vi "国弘恢复出厂.vi"(7 "探头":u16(ring)=5 items=["NULL", "pH", "Cond", "DO", "Turb", "ORP", "6", "7", "8", "9", "氯化物"], 8 "error in (no error)":errorcluster caption="错误输入（无错误）") -> (0 "error out":errorcluster caption="错误输出", 3 "MB session out":refnum<class "MB_Master.lvclass">)   [LabVIEW 2022 SP3, in "斯坦道多参数.lvlib"]
uses:
  <vilib>/Plasmionique/MB Master/MB_Master/MB_Master.lvclass
  <vilib>/Plasmionique/MB Master/MB Master.lvlib
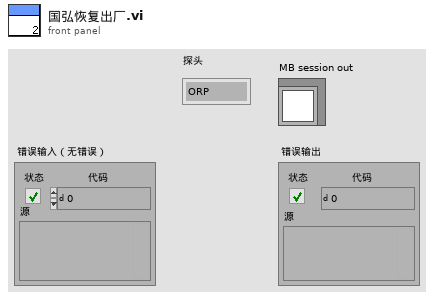
[diagram p1: front panel]
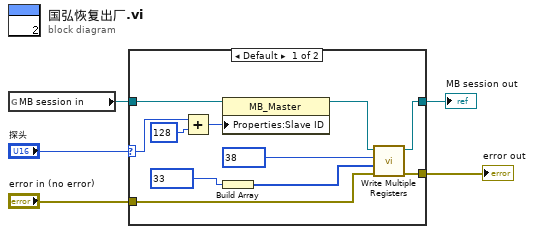
[diagram p0: block diagram]
diagram:
  n1 = global read "多参数全局变量.vi" "MB session in"() -> (w1:refnum<class "MB_Master.lvclass">)
  n2 = case shown="Default" "探头" {
    selector: "探头" -> [w8 _]
    tunnel: "error in (no error)" -> [w15 w17]
    tunnel: w1 -> [w11 w18]
    tunnel: [w10 w17] -> w4
    tunnel: [w9 w18] -> w3
    frame Default {
      n3 = Add(x=w8, y=u16 128) -> (x+y=w14:u16)
      n4 = property class="MB_Master"(reference=w11, "Properties:Slave ID"=w14) -> (reference out=w12:refnum<class "MB_Master.lvclass">)  [unwired: 1 in, 1 out]
      n5 = Build Array(u16 33 ("starting address")) -> (w6:u16[])
      n6 = call <vilib>:"Write Multiple Registers.vi"("error in (no error)"=w15, "values"=w6, "starting address"=u16 38, "MB session in"=w12) -> ("error out"=w10:errorcluster, "MB session out"=w9:refnum<class "MB_Master.lvclass">)  [unwired: 6 in]
    }
    frame 0 {
    }
  }
  "error out" <- w4
  "MB session out" <- w3
